vi "Features_SpecPage.vi"(10 "Spec Page Interface":T2, 11 "MetaDataObj in":refnum<class "MetaDataObj.lvclass">) -> (3 "MetaDataObj out":refnum<class "MetaDataObj.lvclass">)   [LabVIEW 2013, in "FixedChannelTBModuleDecideFeatures.lvclass"]
uses:
  FixedChannelTBModuleDecideFeatures.lvclass
  <resource>/dialog/NewProjectWizard/Spec Page Interface.ctl
  <resource>/dialog/NewProjectWizard/MetaDataObj/MetaDataObj.lvclass
  <resource>/dialog/NewProjectWizard/MetaDataObj/MetaDataObj.lvclass/MetaDataObj.ctl
  FixedChannelTBModuleDecideFeatures.lvclass/FixedChannelTBModuleDecideFeatures.ctl
  <resource>/dialog/NewProjectWizard/MetaDataObj/Accessors/Write Project Name.vi
  <resource>/dialog/NewProjectWizard/MetaDataObj/Accessors/Write Project Root.vi
  Write component name.vi
  Write instances allowed.vi
  <resource>/dialog/NewProjectWizard/MetaDataObj/Accessors/Write File Prefix.vi
panel:
  in  "Tab Control":T1(tab)
  in  "Path to User VI":path
  in  "Instances Allowed":i32=-1
  in  "Module Name":string
  in  "Project Root":path
  # "#TODO Add description"
  # "Execution Behaviors:"
  # "Number of classes allowed in a system. Default is infinite, -1. Examples: {Scaling: -1};{Scan Engine: 1}"
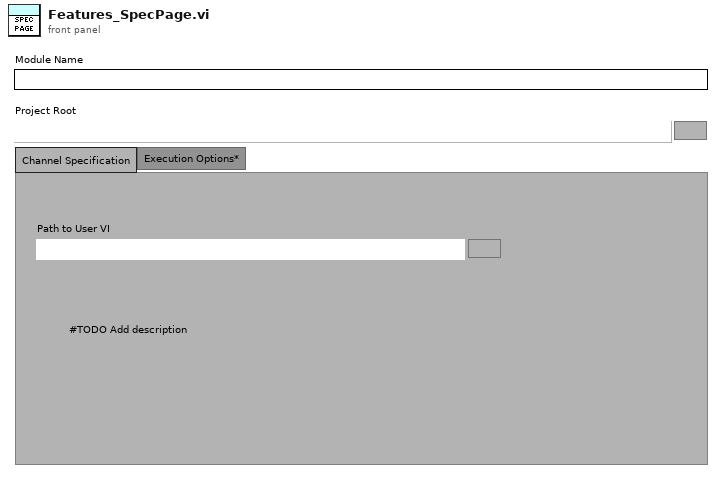
[diagram p1: front panel]
types:
  T1 = enum32{"Channel Specification", "Execution Options*"}
  T2 = typedef "Spec Page Interface.ctl" = cluster{"\"Tab Forward To\" Refnum":refnum<vi>, "\"Tab Backward To\" Refnum":refnum<vi>, "Errors":refnum<user-event>, "Quit":refnum<user-event>}
  T3 = typedef "FixedChannelTBModuleDecideFeatures.lvclass/channel configuration.ctl" = cluster{"Name":string, "channel classification":T4, "data type":T5}
  T4 = typedef "TBM channel.lvclass/channel classification.ctl" = enum16{"input data", "output data", "processing parameter", "processing result"}
  T5 = typedef "tag bus.lvlib/tag descriptor.lvclass/Data Type.ctl" = enum16{"Double", "Single", "I64", "I32", "I16", "I8", "U64", "U32", "U16", "U8", "Boolean", "String", "Array of Double", "Array of Single", "Array of I64", "Array of I32", "Array of I16", "Array of I8", "Array of U64", "Array of U32", "Array of U16", "Array of U8", "Array of Boolean", "Array of String"}
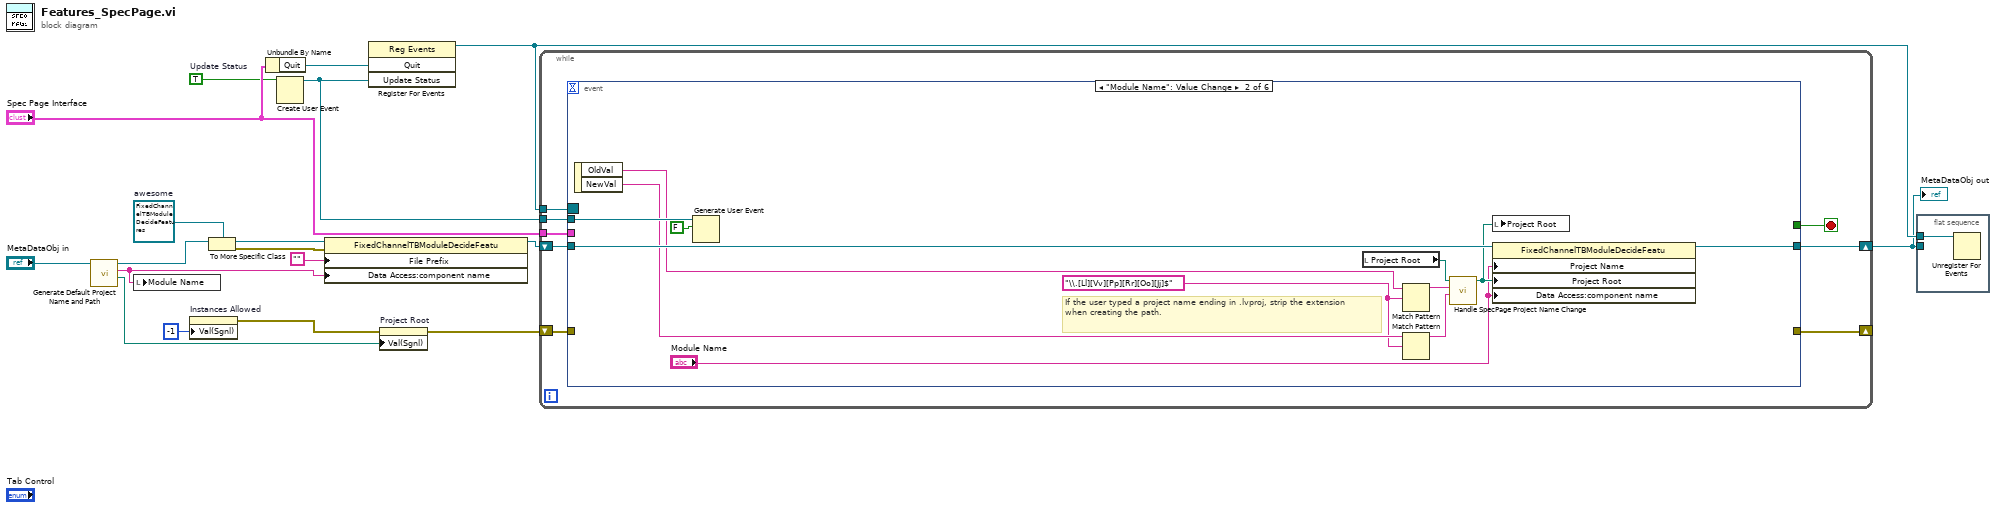
[diagram p0: block diagram]
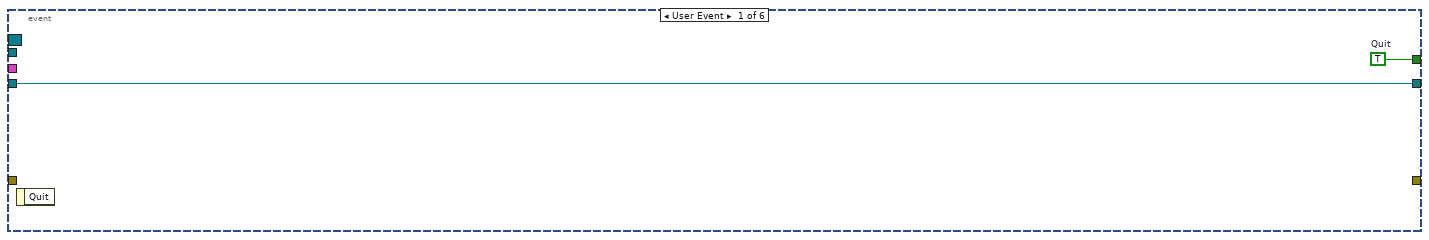
[diagram p2: hidden frame]
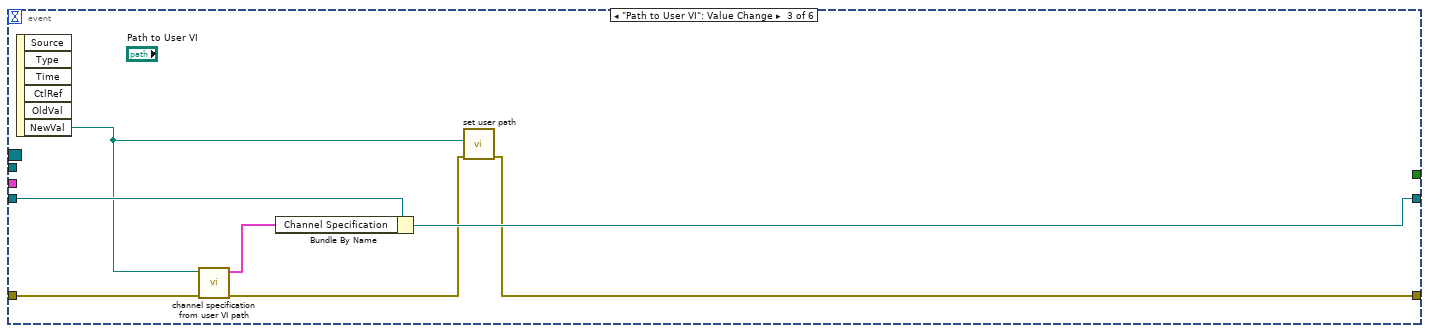
[diagram p3: hidden frame]
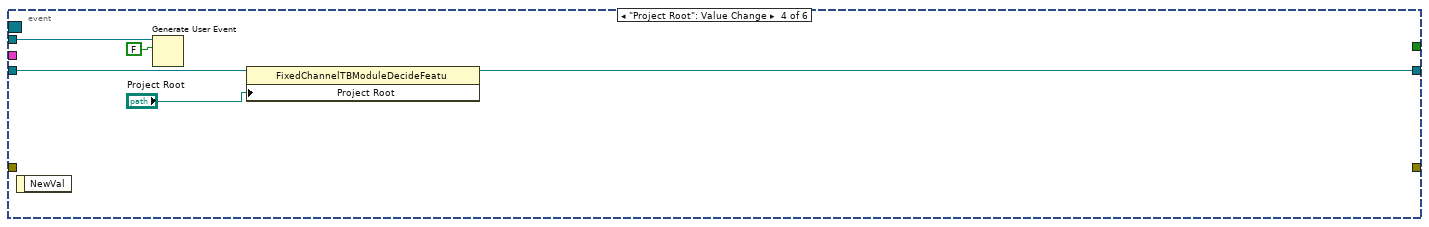
[diagram p4: hidden frame]
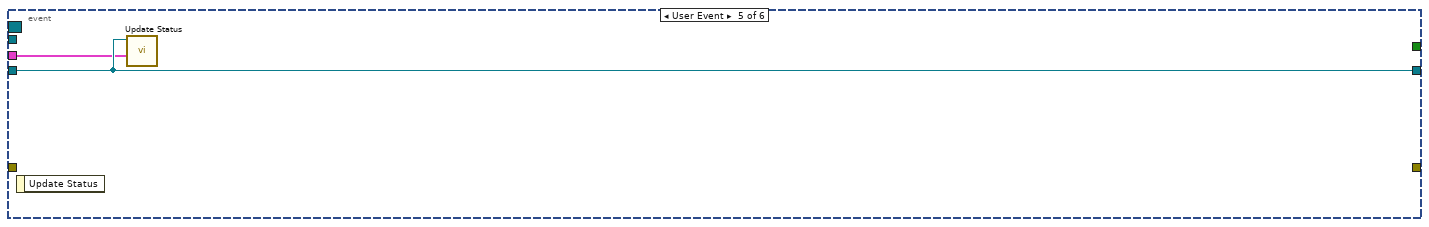
[diagram p5: hidden frame]
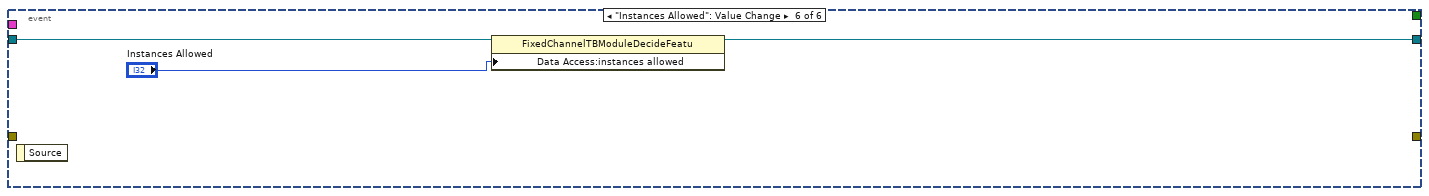
[diagram p6: hidden frame]
diagram:
  w12 = TRUE  # Update Status
  w13 = refnum<class "FixedChannelTBModuleDecideFeatures.lvclass"> refnum  # awesome
  n1 = call <resource>:"Generate Default Project Name and Path.vi"("DNL_MetaDataObj in"="MetaDataObj in") -> ("Project Root"=w5:path, "Project Name"=w3:string, "DNL_MetaDataObj out"=w6:refnum<class "MetaDataObj.lvclass">)  [unwired: 8 in]
  n2 = local write "Module Name"(w3) -> ()
  n3 = property on="Instances Allowed" class="DigNum (strict)"("Val(Sgnl)"=-1 ("Value (Signaling)")) -> (error out=w2:errorcluster)  [unwired: 2 in, 1 out]
  n4 = To More Specific Class(target class=w13, reference=w6) -> (specific class reference=w15:refnum<class "FixedChannelTBModuleDecideFeatures.lvclass">, error out=w14:errorcluster)  [unwired: 1 in]
  n5 = Unbundle By Name("Spec Page Interface") -> ("Quit"=w18:refnum<user-event>)
  n6 = Create User Event(user event datatype=w12) -> (user event=w9:refnum<user-event>)  [unwired: 1 in, 1 out]
  n7 = property class="FixedChannelTBModuleDecideFeatu"(reference=w15, error in=w14, "File Prefix"="", "Data Access:component name"=w3) -> (reference out=w11:refnum<class "FixedChannelTBModuleDecideFeatures.lvclass">)  [unwired: 1 out]
  n8 = register-events(w18, w9) -> (reference out=w17:refnum<event-registration>)  [unwired: 2 in, 1 out]
  n9 = property on="Project Root" class="Path"(error in=w2, "Val(Sgnl)"=w5) -> (error out=w10:errorcluster)  [unwired: 1 in, 1 out]
  n10 = while {
    tunnel: "Spec Page Interface" -> [w25]
    shift-right: [w23] -> w4
    shift-left: w11 -> [w22]
    tunnel: w17 -> [w24]
    tunnel: w9 -> [w21]
    shift-right: [w19] -> _
    shift-left: w10 -> [w20]
    stop <- w26 stop-if-true
    n11 = event shown="[1] \"Module Name\": Value Change" {
      selector: w24 -> [_ _ _ _ _ _]
      dyn-events: _ -> [_ _ _ _ _ _]
      timeout: _ -> [_ _ _ _ _ _]
      tunnel: w25 -> [_ _ _ _ w53 _]
      tunnel: [w28 _ _ _ _ _] -> w26
      tunnel: [w27 w40 w46 w51 w54 w56] -> w23
      tunnel: w22 -> [w27 w37 w47 w52 w54 w57]
      tunnel: w21 -> [_ w39 _ w50 _ _]
      tunnel: w20 -> [_ _ w44 _ _ _]
      tunnel: [_ _ w41 _ _ _] -> w19
      event User Event {
        w28 = TRUE  # Quit
        n12 = event-data() -> ()  [unwired: 1 in, 1 out]
      }
      event "Module Name": Value Change {
        w32 = "\\.[Ll][Vv][Pp][Rr][Oo][Jj]$" ("regular expression")
        # "If the user typed a project name ending in .lvproj, strip the extension when creating the path."
        n13 = event-data() -> ("OldVal"=w34:string, "NewVal"=w33:string)  [unwired: 1 in]
        n14 = Generate User Event(user event=w39, event data cluster=FALSE ("Update Status")) -> ()  [unwired: 2 in, 2 out]
        n15 = local read "Project Root"() -> (w36:path)
        n16 = Match Pattern(string=w34, regular expression=w32) -> (before substring=w31:string)  [unwired: 1 in, 3 out]
        n17 = Match Pattern(string=w33, regular expression=w32) -> (before substring=w30:string)  [unwired: 1 in, 3 out]
        n18 = call <resource>:"Handle SpecPage Project Name Change.vi"("Project Name New Value"=w30, "Project Name Old Value"=w31, "Project Root in"=w36) -> ("Project Root out"=w35:path)  [unwired: 8 in]
        n19 = local write "Project Root"(w35) -> ()
        n20 = property class="FixedChannelTBModuleDecideFeatu"(reference=w37, "Project Name"="Module Name", "Project Root"=w35, "Data Access:component name"="Module Name") -> (reference out=w40:refnum<class "FixedChannelTBModuleDecideFeatures.lvclass">)  [unwired: 1 in, 1 out]
      }
      event "Path to User VI": Value Change {
        n21 = event-data() -> ("NewVal"=w43:path)  [unwired: 1 in, 5 out]
        n22 = call "channel specification from user VI path.vi"("error in (no error)"=w44, "User VI Path in"=w43) -> ("error out"=w42:errorcluster, "Channel Specification out"=w45:T3[])  [unwired: 8 in]
        n23 = Bundle By Name(cluster=w47, "Channel Specification"=w45) -> (w46:refnum<class "FixedChannelTBModuleDecideFeatures.lvclass">)
        n24 = call "set user path.vi"("error in (no error)"=w42, "User VI Path"=w43) -> ("error out"=w41:errorcluster)  [unwired: 9 in]
      }
      event "Project Root": Value Change {
        n25 = event-data() -> ()  [unwired: 1 in, 1 out]
        n26 = Generate User Event(user event=w50, event data cluster=FALSE ("Update Status")) -> ()  [unwired: 2 in, 2 out]
        n27 = property class="FixedChannelTBModuleDecideFeatu"(reference=w52, "Project Root"="Project Root") -> (reference out=w51:refnum<class "FixedChannelTBModuleDecideFeatures.lvclass">)  [unwired: 1 in, 1 out]
      }
      event User Event {
        n28 = event-data() -> ()  [unwired: 1 in, 1 out]
        n29 = call "Update Status.vi"("Spec Page Interface"=w53, "TwoTasksMetaDataObj in"=w54) -> ()  [unwired: 10 in]
      }
      event "Instances Allowed": Value Change {
        n30 = event-data() -> ()  [unwired: 1 in, 1 out]
        n31 = property class="FixedChannelTBModuleDecideFeatu"(reference=w57, "Data Access:instances allowed"="Instances Allowed") -> (reference out=w56:refnum<class "FixedChannelTBModuleDecideFeatures.lvclass">)  [unwired: 1 in, 1 out]
      }
    }
  }
  "MetaDataObj out" <- w4
  n32 = flat-sequence {
    tunnel: w17 -> [w58]
    tunnel: w4 -> [_]
    frame #0 {
      n33 = Unregister For Events(event registration refnum=w58) -> ()  [unwired: 1 in, 1 out]
    }
  }
